vi "Stacking Test Pt 2.vi"() -> ()   [LabVIEW 2014]
uses:
  Subsystems VIs/Robot Commands.ctl
  Subsystems VIs/Stacking SS/Stacking SS State.ctl
  Subsystems VIs/Stacking SS/Stacking SS Actuators.ctl
  <vilib>/Rock Robotics/WPI/Solenoid/WPI_SolenoidValue.ctl
  Global Variables/Sensor Data (Edited).vi
  Global Variables/Miscalleneous.vi
  Global Variables/Settings.vi
  Global Variables/Lifter Sequences.vi
panel:
  out "Totes in Bot":i32
  in  "Slide":dbl(slide) scale=0.0..36.125
  out "Stacking Actuators Out":T1
  in  "Stacking SS State":T3
  in  "Robot Controls":T4
  in  "Scissors Deployment finished":bool
  in  "Tote in Position/Ready to Stack":bool
  out "Lift Position 5":bool
  out "Lift Position 4":bool
  out "Lift Position 3":bool
  out "Lift Position 2":bool
  out "Lift Position 1":bool
  # "Field Centric"
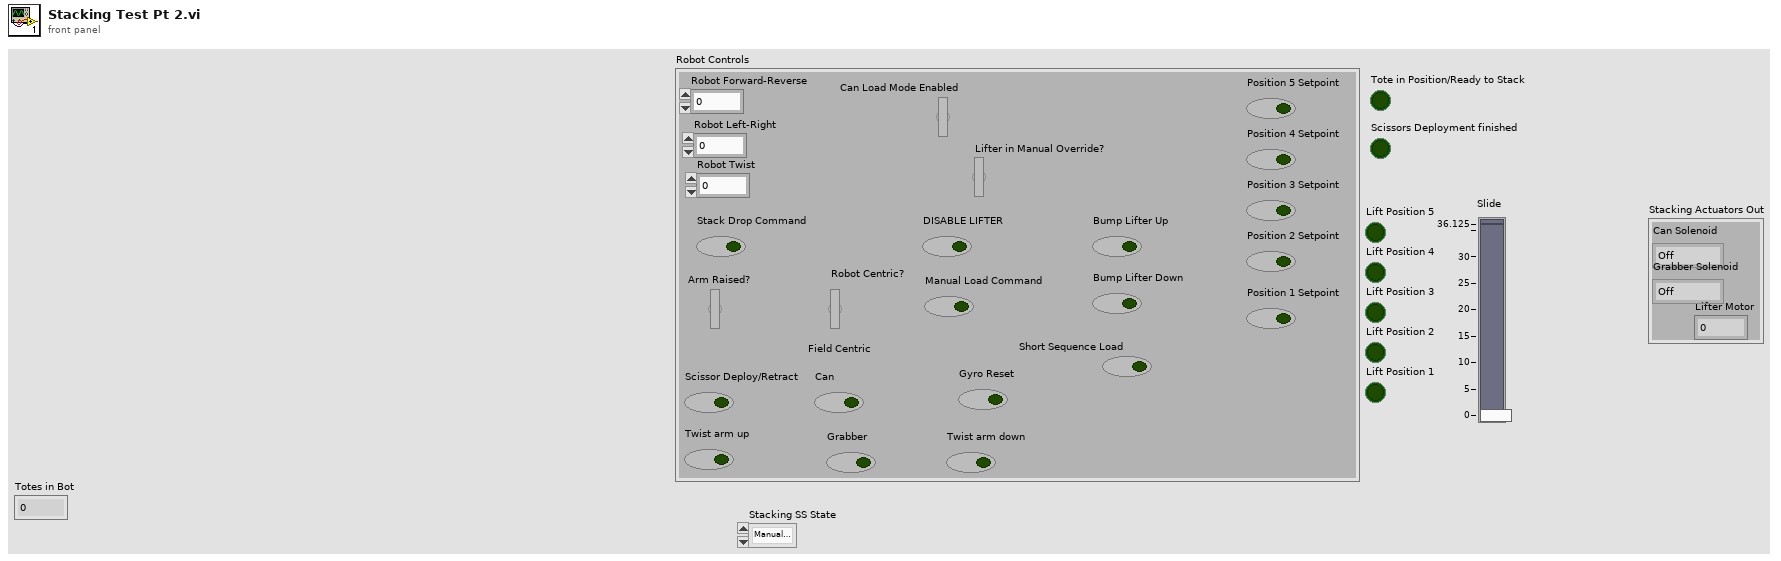
[diagram p1: front panel]
types:
  T1 = typedef "Stacking SS Actuators.ctl" = cluster{"Can Solenoid":T2, "Lifter Motor":dbl, "Grabber Solenoid":T2}
  T2 = typedef "WPI_SolenoidValue.ctl" = enum16{"Off", "On", "Forward", "Reverse"}
  T3 = typedef "Stacking SS State.ctl" = enum16{"Manual Load", "Manual Override"}
  T4 = typedef "Robot Commands.ctl" = cluster{"Robot Forward-Reverse":dbl, "Robot Left-Right":dbl, "Robot Twist":dbl, "Can Load Mode Enabled":bool, "Lifter in Manual Override?":bool, "Stack Drop Command":bool, "Arm Raised?":bool, "DISABLE LIFTER":bool, "Position 1 Setpoint":bool, "Position 2 Setpoint":bool, "Position 3 Setpoint":bool, "Position 4 Setpoint":bool, "Position 5 Setpoint":bool, "Bump Lifter Down":bool, "Bump Lifter Up":bool, "Manual Load Command":bool, "Robot Centric?":bool, "Scissor Deploy/Retract":bool, "Grabber":bool, "Can":bool, "Twist arm up":bool, "Gyro Reset":bool, "Twist arm down":bool, "Short Sequence Load":bool}
  T5 = cluster{"Setpoint Commands":enum16{"No Op", "Setpoint 1", "Setpoint 2", "Setpoint 3", "Setpoint 4", "Setpoint 5"}[], "Setpoint Commands Wait for Input?":bool[], "Setpoint Commands Time Wait after setpoint reachd":i32[], "Can Solenoid Commands":enum16{"Disengaged", "Engaged"}[], "Grabber Solenoid Commands":enum16{"Disengaged", "Engaged"}[]}
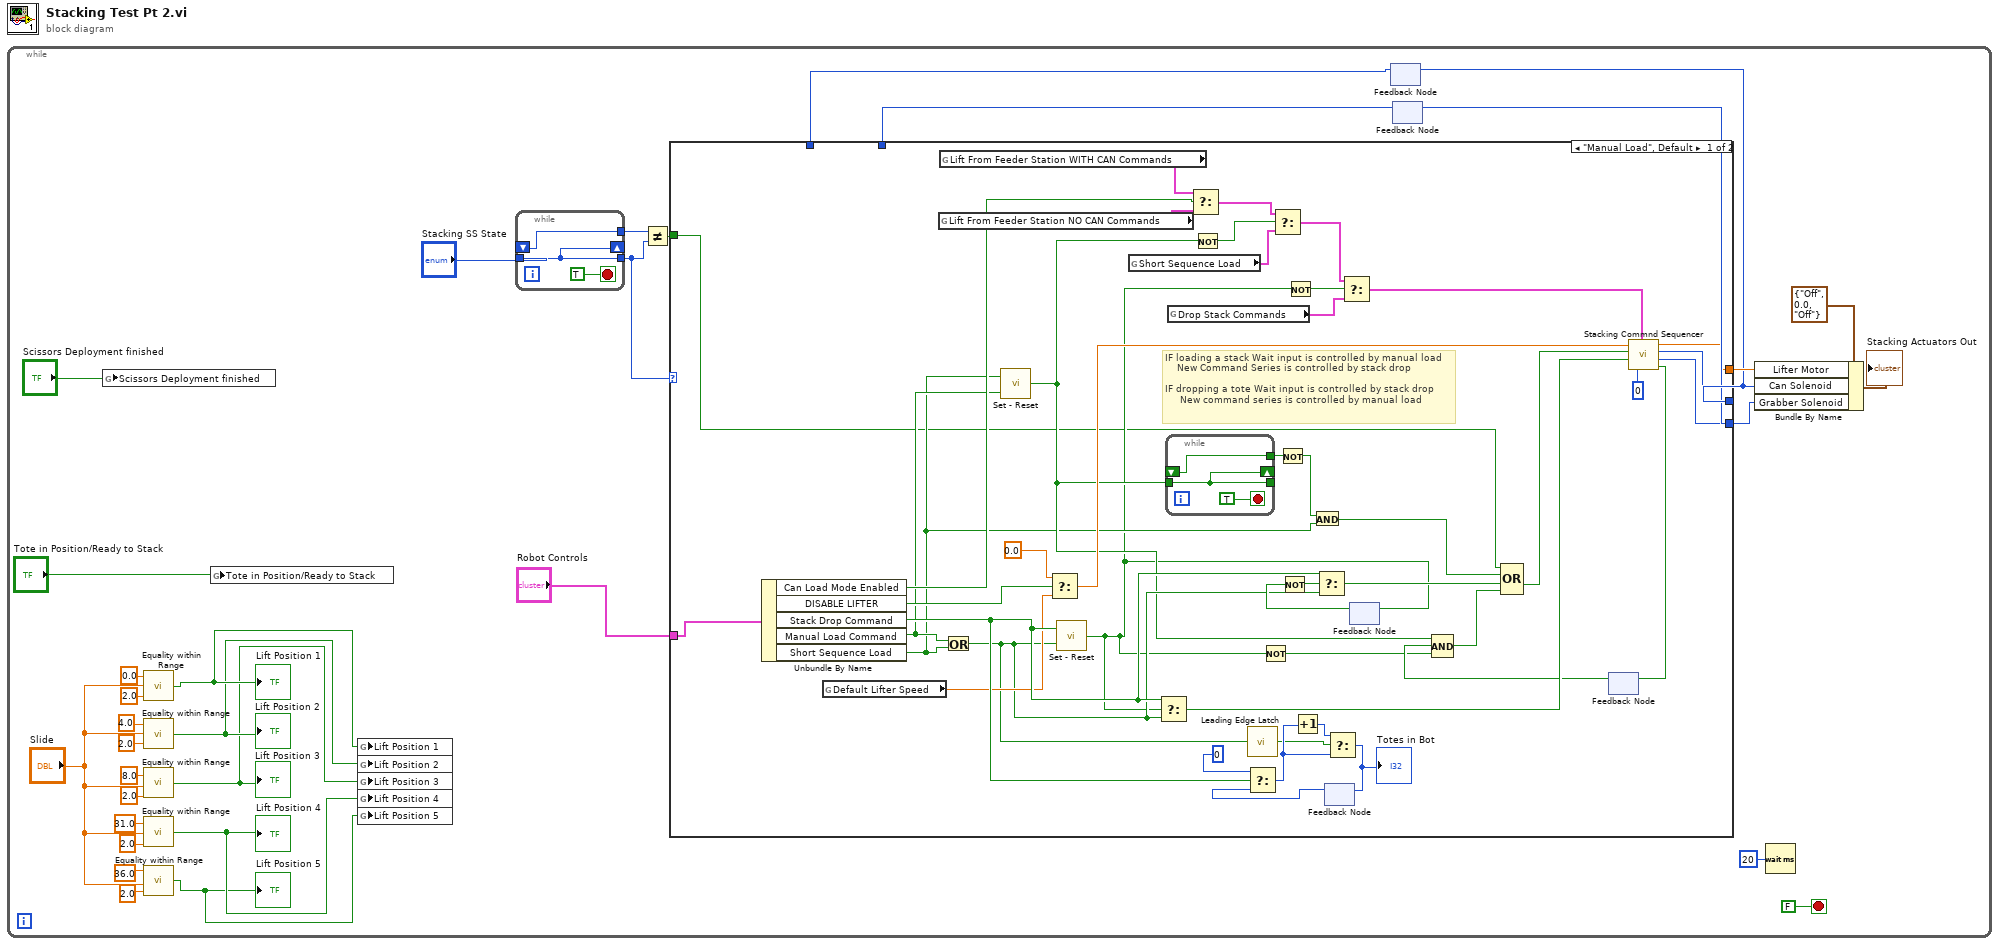
[diagram p0: block diagram]
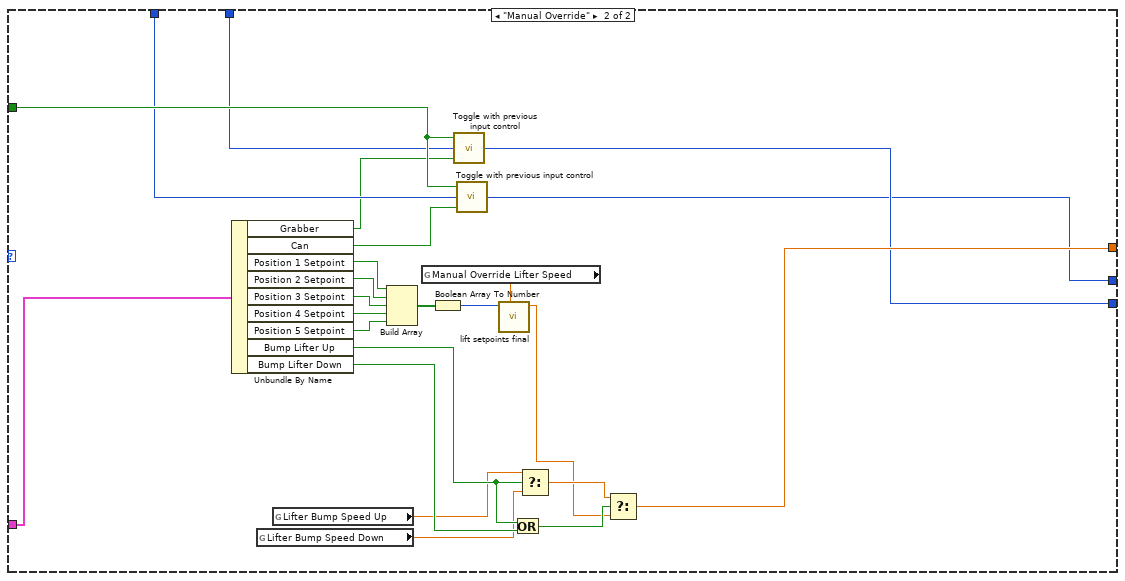
[diagram p2: hidden frame]
diagram:
  n1 = while {
    stop <- FALSE stop-if-true
    n2 = global write "Miscalleneous.vi" "Scissors Deployment finished"("Scissors Deployment finished") -> ()
    n3 = call "Equality within Range.vi"("Range"=2.0, "Y"="Slide", "X"=0.0) -> ("X = Y within Range?"=w9:bool)
    "Lift Position 1" <- w9
    n4 = call "Equality within Range.vi"("Range"=2.0, "Y"="Slide", "X"=4.0) -> ("X = Y within Range?"=w8:bool)
    "Lift Position 2" <- w8
    n5 = call "Equality within Range.vi"("Range"=2.0, "Y"="Slide", "X"=8.0) -> ("X = Y within Range?"=w7:bool)
    "Lift Position 3" <- w7
    n6 = call "Equality within Range.vi"("Range"=2.0, "Y"="Slide", "X"=31.0) -> ("X = Y within Range?"=w6:bool)
    "Lift Position 4" <- w6
    n7 = call "Equality within Range.vi"("Range"=2.0, "Y"="Slide", "X"=36.0) -> ("X = Y within Range?"=w5:bool)
    "Lift Position 5" <- w5
    n8 = global write "Sensor Data (Edited).vi" "Tote in Position/Ready to Stack"("Tote in Position/Ready to Stack") -> ()
    n9 = global write "Sensor Data (Edited).vi" "Lift Position 1"(w9) -> ()
    n10 = global write "Sensor Data (Edited).vi" "Lift Position 2"(w8) -> ()
    n11 = global write "Sensor Data (Edited).vi" "Lift Position 3"(w7) -> ()
    n12 = global write "Sensor Data (Edited).vi" "Lift Position 4"(w6) -> ()
    n13 = global write "Sensor Data (Edited).vi" "Lift Position 5"(w5) -> ()
    n14 = while {
      tunnel: "Stacking SS State" -> [w105]
      tunnel: [w105] -> w21
      shift-right: [w105] -> _
      shift-left: _ -> [w104]
      tunnel: [w104] -> w22
      stop <- TRUE stop-if-true
    }
    n15 = Not Equal?(x=w22, y=w21) -> (x != y?=w23:bool)
    n16 = feedback #1() -> (w3:T2)  [unwired: 1 in]
    n17 = feedback #2() -> (w1:T2)  [unwired: 1 in]
    n18 = case shown="\"Manual Load\", Default" w21 {
      tunnel: "Robot Controls" -> [w37 w88]
      tunnel: [w33 w87] -> w24
      tunnel: w23 -> [w36 w86]
      tunnel: [w34 w80] -> w4
      tunnel: [w35 w81] -> w2
      tunnel: w3 -> [_ w83]
      tunnel: w1 -> [_ w85]
      frame "Manual Load", Default {
        # "IF loading a stack Wait input is controlled by manual load\n    New Command Series is controlled by stack drop\n\nIF dropping a tote Wait input is controlled by stack drop\n     New command series is controlled by manual load"
        n19 = Unbundle By Name(w37) -> ("Can Load Mode Enabled"=w73:bool, "DISABLE LIFTER"=w75:bool, "Stack Drop Command"=w71:bool, "Manual Load Command"=w46:bool, "Short Sequence Load"=w43:bool)
        n20 = global read "Settings.vi" "Default Lifter Speed"() -> (w69:dbl)
        n21 = global read "Lifter Sequences.vi" "Lift From Feeder Station NO CAN Commands"() -> (w62:T5)
        n22 = global read "Lifter Sequences.vi" "Lift From Feeder Station WITH CAN Commands"() -> (w61:T5)
        n23 = Or(x=w46, y=w43) -> (x .or. y?=w54:bool)
        n24 = call "Set - Reset.vi"("Reset"=w46, "Set"=w43) -> ("Output"=w44:bool)
        n25 = Select(t=0.0 ("Set Motor Speed"), s=w75, f=w69) -> (s? t:f=w74:dbl)
        n26 = call "Set - Reset.vi"("Reset"=w54, "Set"=w71) -> ("Output"=w40:bool)
        n27 = global read "Lifter Sequences.vi" "Short Sequence Load"() -> (w51:T5)
        n28 = Select(t=w71, s=w40, f=w54) -> (s? t:f=w50:bool)
        n29 = while {
          tunnel: w44 -> [w78]
          tunnel: [w78] -> _
          shift-right: [w78] -> _
          shift-left: _ -> [w77]
          tunnel: [w77] -> w42
          stop <- TRUE stop-if-true
        }
        n30 = global read "Lifter Sequences.vi" "Drop Stack Commands"() -> (w59:T5)
        n31 = Select(t=w61, s=w73, f=w62) -> (s? t:f=w52:T5)
        n32 = Not(x=w44) -> (.not. x?=w45:bool)
        n33 = call "Leading Edge Latch.vi"("Input"=w54) -> ("Output"=w57:bool)
        n34 = Not(x=w40) -> (.not. x?=w39:bool)
        n35 = Select(t=w52, s=w45, f=w51) -> (s? t:f=w53:T5)
        n36 = Not(x=w42) -> (.not. x?=w41:bool)
        n37 = Not(x=w40) -> (.not. x?=w58:bool)
        n38 = And(x=w41, y=w43) -> (x .and. y?=w38:bool)
        n39 = feedback #3() -> (w64:i32)  [unwired: 1 in]
        n40 = Select(t=0, s=w71, f=w64) -> (s? t:f=w66:i32)
        n41 = Increment(x=w66) -> (x+1=w67:i32)
        n42 = Select(t=w67, s=w57, f=w66) -> (s? t:f=w65:i32)
        "Totes in Bot" <- w65
        n43 = feedback-in #3(w65) -> ()
        n44 = Select(t=w53, s=w58, f=w59) -> (s? t:f=w70:T5)
        n45 = feedback #4() -> (w56:bool)  [unwired: 1 in]
        n46 = Not(x=w56) -> (.not. x?=w55:bool)
        n47 = Select(t=w71, s=w55, f=w54) -> (s? t:f=w60:bool)
        n48 = feedback-in #4(w40) -> ()
        n49 = feedback #5() -> (w48:bool)  [unwired: 1 in]
        n50 = Compound Arithmetic op=AND(w44, w48, w39) -> (w47:bool)
        n51 = Compound Arithmetic op=OR(w36, w38, w60, w47) -> (w72:bool)
        n52 = call "Stacking Commnd Sequencer.vi"("Lifter Commands"=w70, "Command Series Start Index"=0, "Wait Input"=w50, "New Command Series"=w72, "Set Motor Speed"=w74) -> ("Series Finished"=w49:bool, "Grabber Solenoid"=w35:T2, "Can Solenoid"=w34:T2, "Motor Speed"=w33:dbl)
        n53 = feedback-in #5(w49) -> ()
      }
      frame "Manual Override" {
        n54 = Unbundle By Name(w88) -> ("Grabber"=w82:bool, "Can"=w84:bool, "Position 1 Setpoint"=w103:bool, "Position 2 Setpoint"=w102:bool, "Position 3 Setpoint"=w101:bool, "Position 4 Setpoint"=w100:bool, "Position 5 Setpoint"=w99:bool, "Bump Lifter Up"=w97:bool, "Bump Lifter Down"=w96:bool)
        n55 = global read "Settings.vi" "Lifter Bump Speed Down"() -> (w90:dbl)
        n56 = global read "Settings.vi" "Lifter Bump Speed Up"() -> (w91:dbl)
        n57 = Build Array(w103, w102, w101, w100, w99) -> (w98:bool[])
        n58 = global read "Settings.vi" "Manual Override Lifter Speed"() -> (w92:dbl)
        n59 = Boolean Array To Number(Boolean array=w98) -> (number=w89:u32)
        n60 = call "Toggle with previous input control.vi"("Control"=w82, "Previous Input"=w85, "Reset to Previous Input?"=w86) -> ("Output"=w81:T2)
        n61 = call "Toggle with previous input control.vi"("Control"=w84, "Previous Input"=w83, "Reset to Previous Input?"=w86) -> ("Output"=w80:T2)
        n62 = call "lift setpoints final.vi"("Set Motor Speed"=w92, "Requested Position\n(0, 1, 2, 4, 8, 16)"=w89) -> ("Motor Speed"=w93:dbl)  [unwired: 8 in, 1 out]
        n63 = Or(x=w97, y=w96) -> (x .or. y?=w95:bool)
        n64 = Select(t=w91, s=w97, f=w90) -> (s? t:f=w94:dbl)
        n65 = Select(t=w94, s=w95, f=w93) -> (s? t:f=w87:dbl)
      }
    }
    n66 = feedback-in #1(w4) -> ()
    n67 = feedback-in #2(w2) -> ()
    n68 = Bundle By Name(cluster=T1 {"Can Solenoid"=enum."Off", "Lifter Motor"=0.0, "Grabber Solenoid"=enum."Off"} ("Stacking Actuators Out"), "Lifter Motor"=w24, "Can Solenoid"=w4, "Grabber Solenoid"=w2) -> (→"Stacking Actuators Out":T1)
    n69 = Wait (ms)(milliseconds to wait=u32 20) -> ()  [unwired: 1 out]
  }
